vi "Launch Timer Actor.vi"(8 "error in (no error)":errorcluster, 10 "Timer (s)":dbl) -> (0 "error out":errorcluster, 3 "Timer out":refnum<class "Timer.lvclass">)   [LabVIEW 2021, in "Timer.lvlib" / "Timer.lvclass"]
uses:
  Timer.lvclass
  Timer.lvclass/Timer.ctl
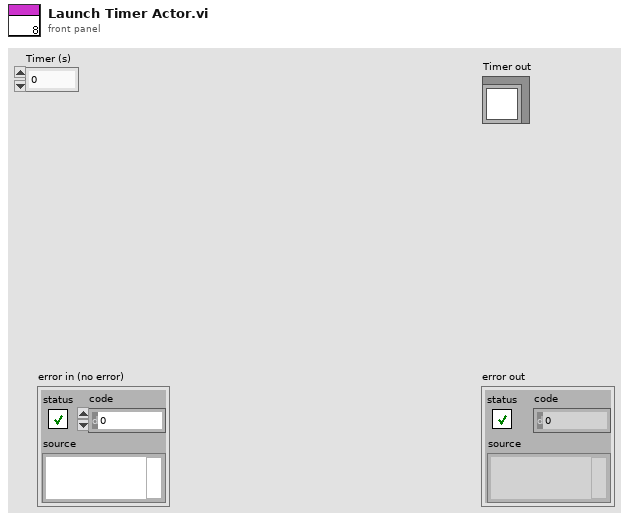
[diagram p1: front panel]
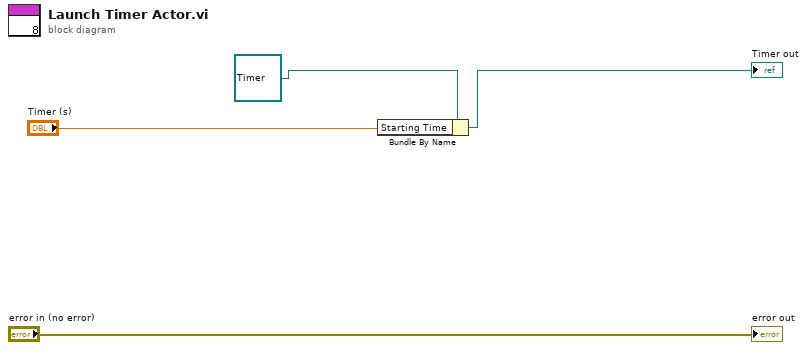
[diagram p0: block diagram]
diagram:
  n1 = Bundle By Name(cluster=refnum<class "Timer.lvclass"> refnum ("Timer out"), "Starting Time"="Timer (s)") -> (→"Timer out":refnum<class "Timer.lvclass">)
  "error out" <- "error in (no error)"
